vi "Variant Decode.vi"(8 "error in (no error)":errorcluster, 11 "variant":variant) -> (0 "error out":errorcluster, 1 "Array Dimensions (Reversed)":i32[](array[numeric]), 3 "Variant Data":T1[](array[typedef]))   [LabVIEW 2011, in "JSON Scalar.lvclass"]
doc: "Decodes compound variant data (clusters array etc) to a list of element data."
uses:
  JSON Scalar.lvclass
  Variant Data Typdef.ctl
  <vilib>/Utility/VariantDataType/Type.ctl
  <vilib>/Utility/VariantDataType/VariantType.lvlib
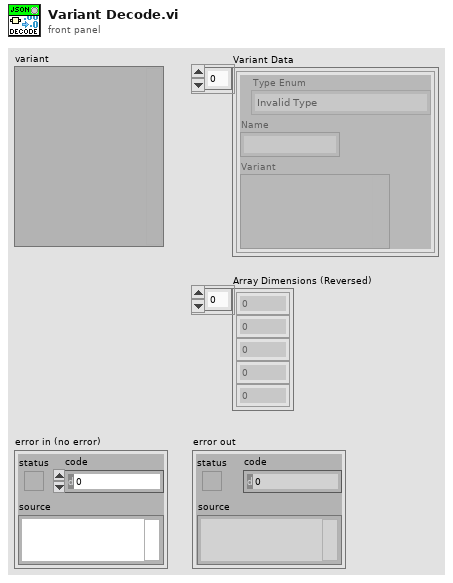
[diagram p1: front panel]
types:
  T1 = typedef "JSON Scalar.lvclass/Variant Data Typdef.ctl" = cluster{"Type Enum":T2, "Name":string, "Variant":variant}
  T2 = typedef "VariantType.lvlib/Type.ctl" = enum8{"Invalid Type", "Void", "I8", "I16", "I32", "I64", "U8", "U16", "U32", "U64", "Single Float", "Double Float", "Extended Float", "Single Complex", "Double Complex", "Extended Complex", "Enum U8", "Enum U16", "Enum U32", "Enum U64", "Single Float With Unit", "Double Float With Unit", "Extended Float With Unit", "Single Complex with Unit", "Double Complex with Unit", "Extended Complex with Unit", "Boolean", "String", "Path", "Picture", "Tag", "Array", "Cluster", "Variant", "LV Variant", "Waveform", "Timestamp", "Digital Waveform", "Digital Data", "ExpressData", "Refnum", "External Data", "VI", "Poly VI", "LabVIEW Class Instance", "Fixed Point"}
  T3 = cluster{"Type":T2, "Element Name":string, "Data":variant}
  T4 = cluster{"Type":T2, "Element Name":string, "Data":variant}[]
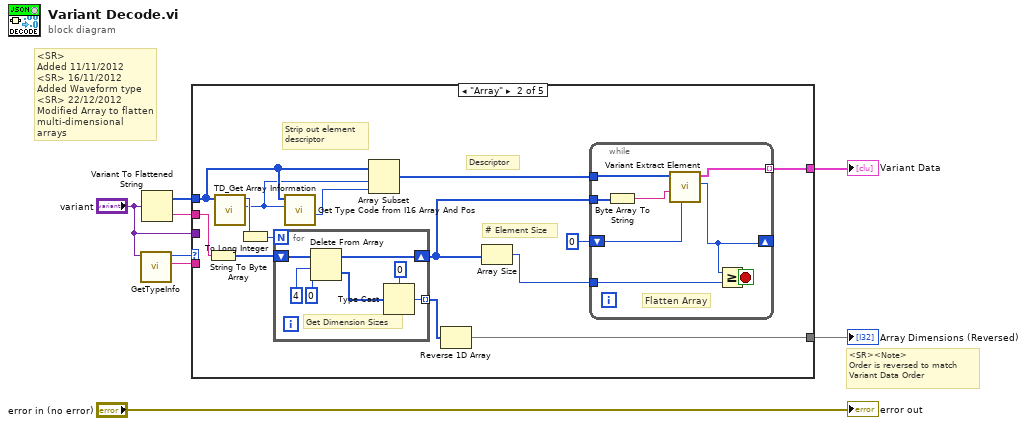
[diagram p0: block diagram]
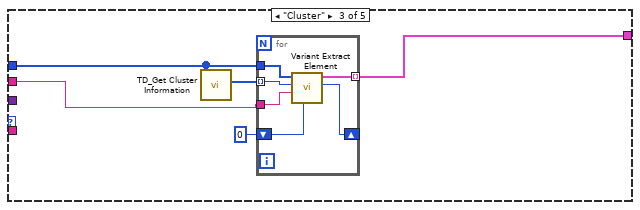
[diagram p3: hidden frame]
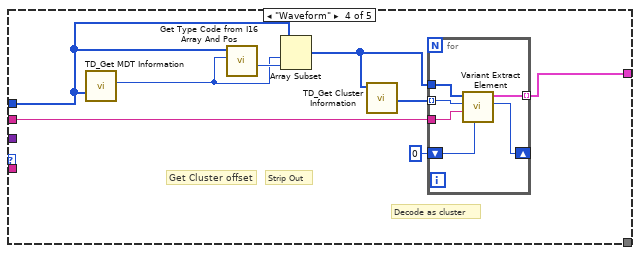
[diagram p4: hidden frame]
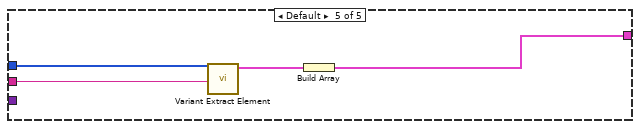
[diagram p5: hidden frame]
diagram:
  # "<SR><Note>\nOrder is reversed to match\nVariant Data Order"
  # "<SR>\nAdded 11/11/2012\n<SR> 16/11/2012\nAdded Waveform type\n<SR> 22/12/2012\nModified Array to flatten\nmulti-dimensional arrays"
  n1 = call <vilib>:"GetTypeInfo.vi"("Variant"="variant") -> ("Name"=w4:string, "Type Enum"=w8:T2)  [unwired: 6 in, 3 out]
  n2 = Variant To Flattened String(Variant="variant") -> (data string=w5:string, 1:w6:i16[])
  n3 = case shown="\"Array\"" w8 {
    tunnel: [_ w11 w40 w54 w63] -> w3
    tunnel: w6 -> [_ w17 w39 w52 w66]
    tunnel: w5 -> [_ w22 w38 w49 w65]
    tunnel: w4 -> [_ _ _ _ _]
    tunnel: "variant" -> [_ _ _ _ _]
    tunnel: [_ w12 _ _ _] -> w1
    frame "Invalid Type", "Void" {
    }
    frame "Array" {
      # "Descriptor"
      # "# Element Size"
      # "Strip out element\ndescriptor"
      n4 = String To Byte Array(string=w22) -> (unsigned byte array=w20:u8[])
      n5 = call <vilib>:"TD_Get Array Information.vi"("Type descriptor"=w17) -> ("Contained TD Offset"=w16:i32, "Number of Dimensions"=w21:i16)  [unwired: 8 in, 1 out]
      n6 = To Long Integer(number=w21) -> (32bit integer=w10:i32)
      n7 = for {
        N: w10 -> [_]
        tunnel: [w32] -> w9 mode=indexing
        shift-right: [w35] -> w14
        shift-left: w20 -> [w37]
        # "Get Dimension Sizes"
        n8 = Delete From Array(array=w37, length=4, index=0) -> (deleted portion=w34:u8[], array with subset deleted=w35:u8[])
        n9 = Type Cast(type=0 ("unsigned 32bit integer"), x=w34) -> (*(type *) &x=w32:i32)
      }
      n10 = call <vilib>:"Get Type Code from I16 Array And Pos.vi"("Pos in Type Descriptor (0)"=w16, "Type descriptor"=w17) -> ("Size (Words)"=w18:i32)  [unwired: 7 in, 2 out]
      n11 = Array Subset(array=w17, index=w16, length=w18) -> (w15:i16[])
      n12 = Reverse 1D Array(array=w9) -> (reversed array=w12:i32[])
      n13 = Array Size(array=w14) -> (size(s)=w13:i32)
      n14 = while {
        tunnel: w15 -> [w28]
        tunnel: w14 -> [w27]
        shift-right: [w24] -> _
        shift-left: 0 -> [w23]
        tunnel: [w25] -> w11 mode=indexing
        tunnel: w13 -> [w29]
        stop <- w30 stop-if-true
        # "Flatten Array"
        n15 = Byte Array To String(unsigned byte array=w27) -> (string=w26:string)
        n16 = call "Variant Extract Element.vi"("Dats Start Pos"=w23, "data string"=w26, "Type Descriptor"=w28) -> ("Data End Pos"=w24:i32, "Element"=w25:T3)  [unwired: 7 in]
        n17 = Greater Or Equal?(x=w24, y=w29) -> (x >= y?=w30:bool)
      }
    }
    frame "Cluster" {
      n18 = call <vilib>:"TD_Get Cluster Information.vi"("Type descriptor"=w39) -> ("Contained TD Offsets"=w42:i32[])  [unwired: 9 in, 1 out]
      n19 = for {
        tunnel: w42 -> [w44] mode=indexing
        tunnel: w38 -> [w47]
        tunnel: w39 -> [w43]
        tunnel: [w48] -> w40 mode=indexing
        shift-right: [w46] -> _
        shift-left: 0 -> [w45]
        n20 = call "Variant Extract Element.vi"("Dats Start Pos"=w45, "data string"=w47, "Descriptor Pos"=w44, "Type Descriptor"=w43) -> ("Data End Pos"=w46:i32, "Element"=w48:T3)  [unwired: 6 in]
      }
    }
    frame "Waveform" {
      # "Decode as cluster"
      # "Strip Out"
      # "Get Cluster offset"
      n21 = call <vilib>:"TD_Get MDT Information.vi"("Type descriptor"=w52) -> ("Contained Cluster Offset"=w51:i32)  [unwired: 9 in, 1 out]
      n22 = call <vilib>:"Get Type Code from I16 Array And Pos.vi"("Pos in Type Descriptor (0)"=w51, "Type descriptor"=w52) -> ("Size (Words)"=w53:i32)  [unwired: 7 in, 2 out]
      n23 = Array Subset(array=w52, index=w51, length=w53) -> (w50:i16[])
      n24 = call <vilib>:"TD_Get Cluster Information.vi"("Type descriptor"=w50) -> ("Contained TD Offsets"=w56:i32[])  [unwired: 9 in, 1 out]
      n25 = for {
        tunnel: w56 -> [w58] mode=indexing
        tunnel: w49 -> [w61]
        tunnel: w50 -> [w57]
        tunnel: [w62] -> w54 mode=indexing
        shift-right: [w60] -> _
        shift-left: 0 -> [w59]
        n26 = call "Variant Extract Element.vi"("Dats Start Pos"=w59, "data string"=w61, "Descriptor Pos"=w58, "Type Descriptor"=w57) -> ("Data End Pos"=w60:i32, "Element"=w62:T3)  [unwired: 6 in]
      }
    }
    frame Default {
      n27 = call "Variant Extract Element.vi"("data string"=w65, "Type Descriptor"=w66) -> ("Element"=w64:T3)  [unwired: 8 in, 1 out]
      n28 = Build Array(w64) -> (w63:T4)
    }
  }
  "Variant Data" <- w3
  "Array Dimensions (Reversed)" <- w1
  "error out" <- "error in (no error)"
